vi "BaudType_CONVERT.vi"(1 "BaudType":T9={"Baud"=0, "SJW"=1, "BRP"=1, "SAM"=0, "PHSEG2_SEL"=0, "PRSEG"=1, "PHSEG1"=1, "PHSEG2"=1} {"PHSEG2" items=["CAN_BIT_1TQ"=1, "CAN_BIT_2TQ"=2, "CAN_BIT_3TQ"=3, "CAN_BIT_4TQ"=4, "CAN_BIT_5TQ"=5, "CAN_BIT_6TQ"=6, "CAN_BIT_7TQ"=7, "CAN_BIT_8TQ"=8]; "PHSEG1" items=["CAN_BIT_1TQ"=1, "CAN_BIT_2TQ"=2, "CAN_BIT_3TQ"=3, "CAN_BIT_4TQ"=4, "CAN_BIT_5TQ"=5, "CAN_BIT_6TQ"=6, "CAN_BIT_7TQ"=7, "CAN_BIT_8TQ"=8]; "PRSEG" items=["CAN_BIT_1TQ"=1, "CAN_BIT_2TQ"=2, "CAN_BIT_3TQ"=3, "CAN_BIT_4TQ"=4, "CAN_BIT_5TQ"=5, "CAN_BIT_6TQ"=6, "CAN_BIT_7TQ"=7, "CAN_BIT_8TQ"=8]; "PHSEG2_SEL" items=["由相位缓冲段1时间决定", "可编程"]; "SAM" items=["采样一次", "采样三次"]; "BRP" items=["1"=1, "2"=2, "3"=3, "4"=4, "5"=5, "6"=6, "7"=7, "8"=8, "9"=9, "10"=10, "11"=11, "12"=12, "13"=13, "14"=14, "15"=15, "16"=16, "17"=17, "18"=18, "19"=19, "20"=20, "21"=21, "22"=22, "23"=23, "24"=24, "25"=25, "26"=26, "27"=27, "28"=28, "29"=29, "30"=30, "31"=31, "32"=32, "33"=33, "34"=34, "35"=35, "36"=36, "37"=37, "38"=38, "39"=39, "40"=40, "41"=41, "42"=42, "43"=43, "44"=44, "45"=45, "46"=46, "47"=47, "48"=48, "49"=49, "50"=50, "51"=51, "52"=52, "53"=53, "54"=54, "55"=55, "56"=56, "57"=57, "58"=58, "59"=59, "60"=60, "61"=61, "62"=62, "63"=63, "64"=64]; "SJW" items=["1TQ"=1, "2TQ"=2, "3TQ"=3, "4TQ"=4]}) -> (0 "BaudType_1":T1={"Baud 0"=0, "Baud 1"=0, "Baud 2"=0, "Baud 3"=0, "SJW"=1, "BRP"=1, "SAM"=0, "PHSEG2_SEL"=0, "PRSEG"=1, "PHSEG1"=1, "PHSEG2"=1} {"PHSEG2" items=["CAN_BIT_1TQ"=1, "CAN_BIT_2TQ"=2, "CAN_BIT_3TQ"=3, "CAN_BIT_4TQ"=4, "CAN_BIT_5TQ"=5, "CAN_BIT_6TQ"=6, "CAN_BIT_7TQ"=7, "CAN_BIT_8TQ"=8]; "PHSEG1" items=["CAN_BIT_1TQ"=1, "CAN_BIT_2TQ"=2, "CAN_BIT_3TQ"=3, "CAN_BIT_4TQ"=4, "CAN_BIT_5TQ"=5, "CAN_BIT_6TQ"=6, "CAN_BIT_7TQ"=7, "CAN_BIT_8TQ"=8]; "PRSEG" items=["CAN_BIT_1TQ"=1, "CAN_BIT_2TQ"=2, "CAN_BIT_3TQ"=3, "CAN_BIT_4TQ"=4, "CAN_BIT_5TQ"=5, "CAN_BIT_6TQ"=6, "CAN_BIT_7TQ"=7, "CAN_BIT_8TQ"=8]; "PHSEG2_SEL" items=["由相位缓冲段1时间决定", "可编程"]; "SAM" items=["采样一次", "采样三次"]; "BRP" items=["1"=1, "2"=2, "3"=3, "4"=4, "5"=5, "6"=6, "7"=7, "8"=8, "9"=9, "10"=10, "11"=11, "12"=12, "13"=13, "14"=14, "15"=15, "16"=16, "17"=17, "18"=18, "19"=19, "20"=20, "21"=21, "22"=22, "23"=23, "24"=24, "25"=25, "26"=26, "27"=27, "28"=28, "29"=29, "30"=30, "31"=31, "32"=32, "33"=33, "34"=34, "35"=35, "36"=36, "37"=37, "38"=38, "39"=39, "40"=40, "41"=41, "42"=42, "43"=43, "44"=44, "45"=45, "46"=46, "47"=47, "48"=48, "49"=49, "50"=50, "51"=51, "52"=52, "53"=53, "54"=54, "55"=55, "56"=56, "57"=57, "58"=58, "59"=59, "60"=60, "61"=61, "62"=62, "63"=63, "64"=64]; "SJW" items=["1TQ"=1, "2TQ"=2, "3TQ"=3, "4TQ"=4]})   [LabVIEW 2018, in "ControlCan.lvlib"]
uses:
  ControlCan.lvlib
  BaudType.ctl
  SJW.ctl
  BRP.ctl
  SAM.ctl
  PHSEG2_SEL.ctl
  PRSEG.ctl
  PHSEG1.ctl
  PHSEG2.ctl
  BaudType_1.ctl
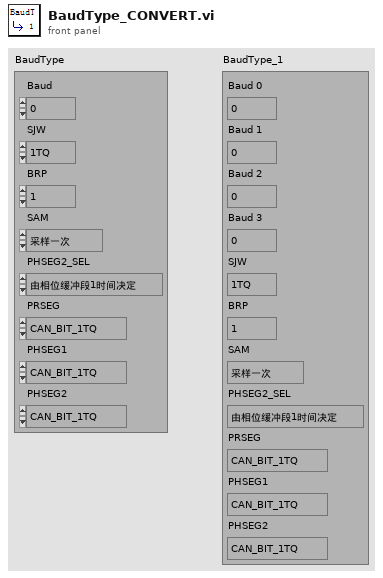
[diagram p1: front panel]
types:
  T1 = typedef "ControlCAN.lvlib/BaudType_1.ctl" = cluster{"Baud 0":u8, "Baud 1":u8, "Baud 2":u8, "Baud 3":u8, "SJW":T2, "BRP":T3, "SAM":T4, "PHSEG2_SEL":T5, "PRSEG":T6, "PHSEG1":T7, "PHSEG2":T8}
  T2 = typedef "ControlCAN.lvlib/SJW.ctl" = u8
  T3 = typedef "ControlCAN.lvlib/BRP.ctl" = u8
  T4 = typedef "ControlCAN.lvlib/SAM.ctl" = u8
  T5 = typedef "ControlCAN.lvlib/PHSEG2_SEL.ctl" = u8
  T6 = typedef "ControlCAN.lvlib/PRSEG.ctl" = u8
  T7 = typedef "ControlCAN.lvlib/PHSEG1.ctl" = u8
  T8 = typedef "ControlCAN.lvlib/PHSEG2.ctl" = u8
  T9 = typedef "ControlCAN.lvlib/BaudType.ctl" = cluster{"Baud":u32, "SJW":T2, "BRP":T3, "SAM":T4, "PHSEG2_SEL":T5, "PRSEG":T6, "PHSEG1":T7, "PHSEG2":T8}
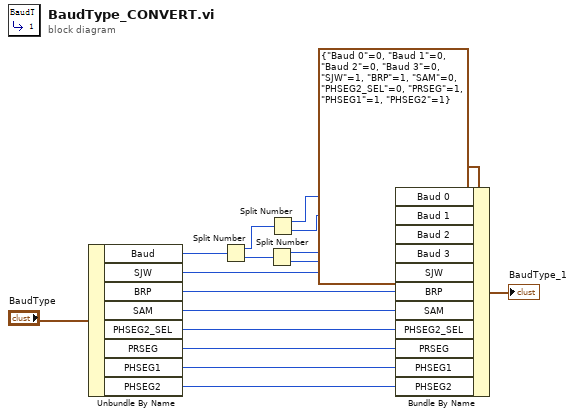
[diagram p0: block diagram]
diagram:
  n1 = Unbundle By Name("BaudType") -> ("Baud"=w15:u32, "SJW"=w8:T2, "BRP"=w7:T3, "SAM"=w6:T4, "PHSEG2_SEL"=w5:T5, "PRSEG"=w4:T6, "PHSEG1"=w3:T7, "PHSEG2"=w2:T8)
  n2 = Split Number(x=w15) -> (hi(x)=w13:u16, lo(x)=w14:u16)
  n3 = Split Number(x=w14) -> (hi(x)=w10:u8, lo(x)=w9:u8)
  n4 = Split Number(x=w13) -> (hi(x)=w12:u8, lo(x)=w11:u8)
  n5 = Bundle By Name(cluster=T1 {"Baud 0"=0, "Baud 1"=0, "Baud 2"=0, "Baud 3"=0, "SJW"=1, "BRP"=1, "SAM"=0, "PHSEG2_SEL"=0, "PRSEG"=1, "PHSEG1"=1, "PHSEG2"=1} ("BaudType_1"), "Baud 0"=w12, "Baud 1"=w11, "Baud 2"=w10, "Baud 3"=w9, "SJW"=w8, "BRP"=w7, "SAM"=w6, "PHSEG2_SEL"=w5, "PRSEG"=w4, "PHSEG1"=w3, "PHSEG2"=w2) -> (→"BaudType_1":T1)
